vi "ATE_ops_cal.vi"() -> ()   [LabVIEW 2012]
doc: "Use this template to build a producer/consumer design pattern with events to produce queue items. Use this design pattern instead of the User Interface Event Handler pattern for user interfaces when you want to execute code asynchronously in response to an event without slowing the user interface responsiveness."
uses:
  Rvp8PowerData.ctl
  <vilib>/Analysis/NI_AALPro.lvlib
panel:
  in  "ABORT":bool
  in  "READY":bool
  out "Instructions":string="rvp8 calibration vi\n\n1 - Disable or turn off transmitter\n2 - Stow Antenna (point vertically)\n3 - Start the labview program by clicking the Run arrow\n     (left most button under  drop down menues)\n     start cycle time about 35 seconds\n3 - Wait for the red 'BUSY' light to change to green 'READY'\n     The 'active' controls on the control tab are the 'TsPring/TsGrabber'\n     and the 'Start dBm', 'Step Size' and 'Steps' controls \n4 - Calibrate with the red  'Calibrate' button\n      calibration cycle time is about 5 minutes\n5 - Calibration cycle can be aborted with the 'Abort Cal' button which\n     is visable only during the cal cycle\n6 - exit the program with the red 'EXIT' button\n      exit cycle time about 20 seconds\n\nHints:\nWait for the green 'READY' light before clicking buttons"
  out "70dB\nAttenuators":bool[](array[boolean])
  out "70 Verfied":bool
  out "121dB\nAttenuators":bool[](array[boolean])
  out "121 Verified":bool
  in  "Configuration 1":bool
  out "Cal Output File":path
  out "Cal differences":cluster{dbl[], dbl[]}[](graph)
  out "RVP8 calibration":cluster{dbl[], dbl[]}[](graph)
  out "Cal file name":string
  in  "Cal data directory":string="/home/spol/projDir/data/cal/ate/rvp8_cal"
  in  "Set SigGen":bool
  in  "Initialize":bool
  in  "70 dB":bool
  in  "121 dB":bool
  in  "Switches":bool
  in  "Calibrate":bool
  in  "Stop":bool
  in  "ATE TABS":enum32{"Status", "Controls"}(tab)=enum."Controls"
  out "ATE Switch Status":T1
  out "RVP8 Power":T2 {"time" format="%<%H:%M:%S\n%Y/%m/%d>T"}
  out "Signal Generator Status":T3={"Frequency (GHz)"=0.0, "RF Power (dBm)"=0.0, "RF Power"=TRUE} {"RF Power (dBm)" format="%.2g"}
  in  "Start dBm":dbl=-14.0 min=-100.0 max=14.0 step=1.0
  in  "Steps":i32=64
  in  "Steps Size":dbl=2.0 min=0.1 max=10.0 step=0.1 format="%.1g"
  in  "121 dB Atten":i32=121 min=0 max=121 step=1
  in  "70 dB Attn":i32=70 min=0 max=70 step=10
  in  "ATE Switches":T4={"Reversing Switch"=enum."Normal Function", "IO Switch #1 Input"=enum."NONE", "IO Switch #1 Output"=enum."NONE", "IO Switch #2 Input"=enum."NONE", "IO Switch #2 Output"=enum."NONE", "Signal Out Input"=enum."NONE", "Signal Out Output"=enum."NONE", "Signal Source Input"=enum."NONE", "Signal Source Output"=enum."NONE", "Power Meter Switch Input"=enum."NONE", "Pouer Meter Switch Output"=enum."NONE", "Amplifier Switch"=enum."Include Amp"}
  in  "DataSource":bool=TRUE
  out "P-State":string
  out "C-State":string
  in  "BUSY":bool
  # "ATE ops cal Program"
  # "10 dB"
  # "20 dB"
  # "40 dB"
  # "1 dB"
  # "2 dB"
  # "4 dB"
  # "4 dB"
  # "10 dB"
  # "20 dB"
  # "40 dB"
  # "40 dB"
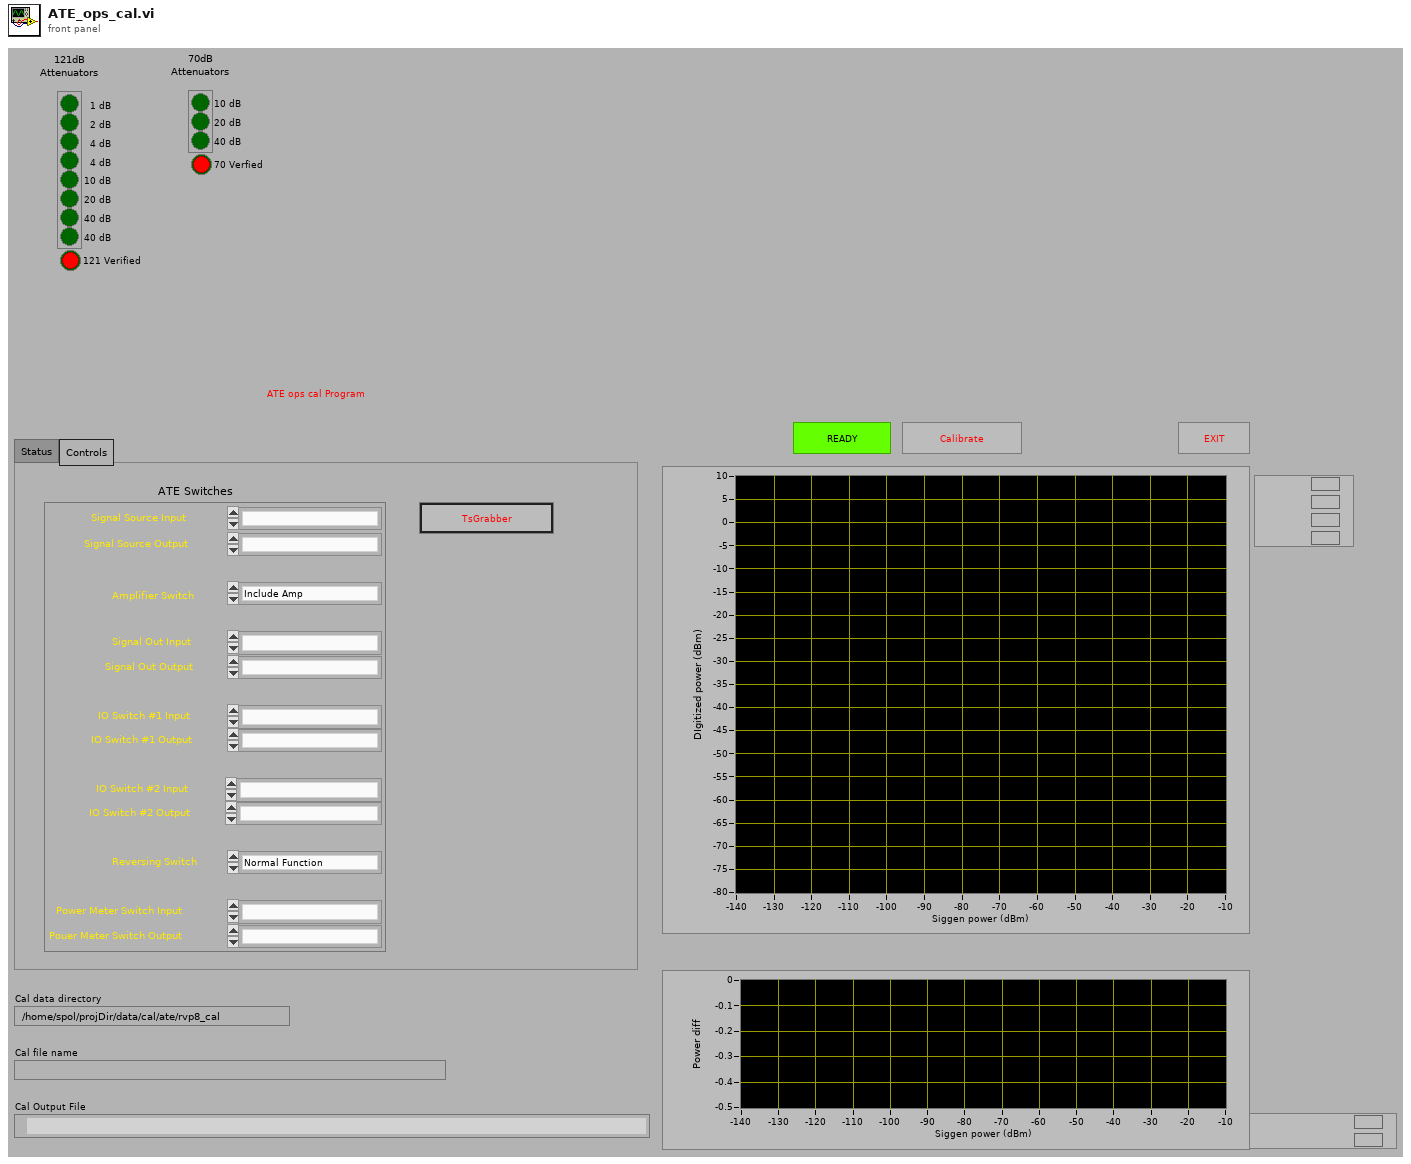
[diagram p1: front panel]
types:
  T1 = cluster{"Reversing Switch ":bool, "IO Switch #1":bool, "IO Switch #2":bool, "Signal Out":bool, "Signal Source":bool, "Power Meter":bool, "Amp By Pass":bool}
  T2 = typedef "Rvp8PowerData.ctl" = cluster{"success":bool, "time":dbl, "el":dbl, "az":dbl, "dbm0":dbl, "dbm1":dbl, "dbmHc":dbl, "dbmHx":dbl, "dbmVc":dbl, "dbmVx":dbl}
  T3 = cluster{"Frequency (GHz)":dbl, "RF Power (dBm)":dbl, "RF Power":bool}
  T4 = cluster{"Reversing Switch":enum16{"Normal Function", "Reversing Function"}, "IO Switch #1 Input":enum16{"NONE", "AHR (J2)", "Splitter", "Signal Out Switch (S3)", "Reversing Switch"}, "IO Switch #1 Output":enum16{"NONE", "AHR (J2)", "Delay Device (S4)", "Power Meter Switch (S5)", "Reversing Switch"}, "IO Switch #2 Input":enum16{"NONE", "AVR (J3)", "Splitter", "Signal Out Switch (S3)", " 2W Term (TM1)", "Reversing Switch"}, "IO Switch #2 Output":enum16{"NONE", "AVR (J3)", "Signal Out Switch (S3)", "Power Meter Switch (S5)", "Reversing Switch", "2W Term (TM1)"}, "Signal Out Input":enum16{"NONE", "Amp Bypass Switch (S6)", "IO Switch #1 (S1)", "IO Switch #2 (S2)", "2W Term (TM3)"}, "Signal Out Output":enum16{"NONE", "2 Watt Term (TM3)", "Splitter", "Power Meter Switch (S5)"}, "Signal Source Input":enum16{"NONE", "Delay Device", "Signal Generator (J7)", "Inside Noise Box NF (J5)", "2W Term (TM3)"}, "Signal Source Output":enum16{"NONE", "Amp Bypass Switch", "Test Pulse Generator", "Power Meter Switch (S5)"}, "Power Meter Switch Input":enum16{"NONE", "IO Switch #1 (S1)", "Signal Source Switch (S4)", "Signal Out Switch (S3)", "IO Switch #2 (S2)", "TXH-TXV Switch (J8)"}, "Pouer Meter Switch Output":enum16{"NONE", "Power Meter (J6)"}, "Amplifier Switch":enum16{"Bypass Amp", "Include Amp"}}
  T5 = cluster{"Frequency (GHz)":dbl, "RF Power (dBm)":dbl, "RF ON/OFF":bool}
  T6 = enum16{"open", "replace", "create", "open or create", "replace or create", "replace or create with confirmation"}
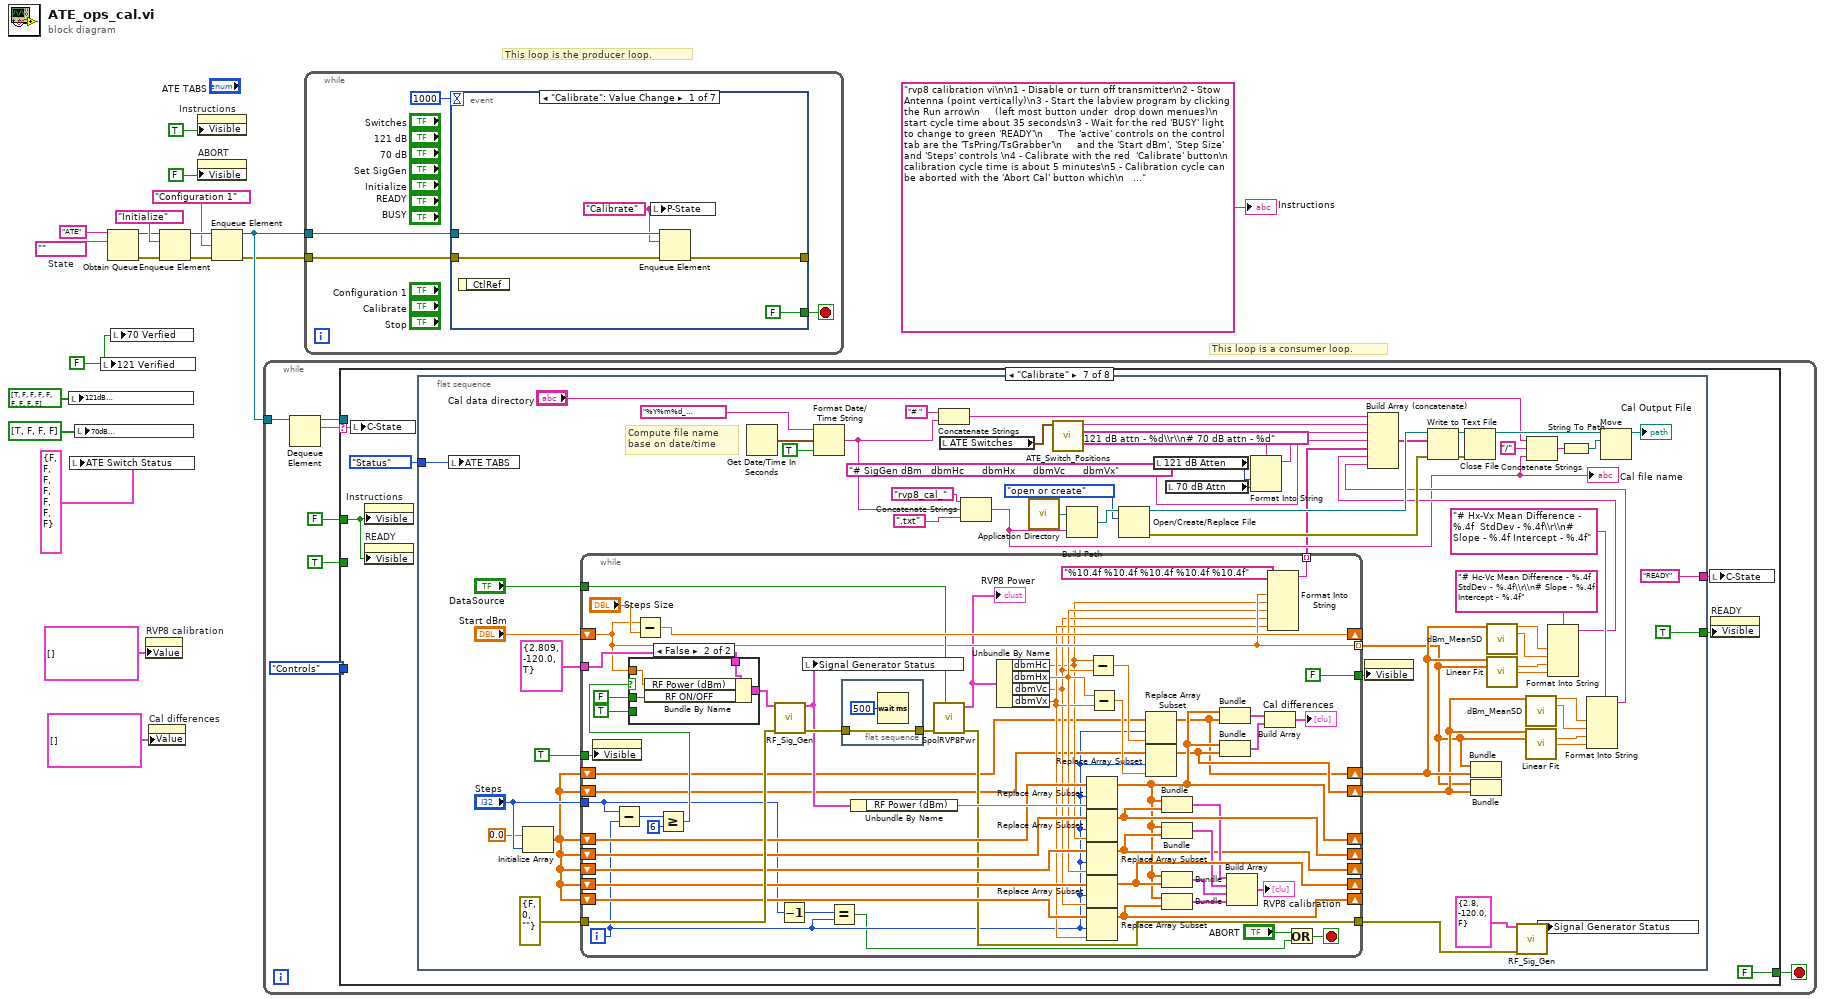
[diagram p0: block diagram]
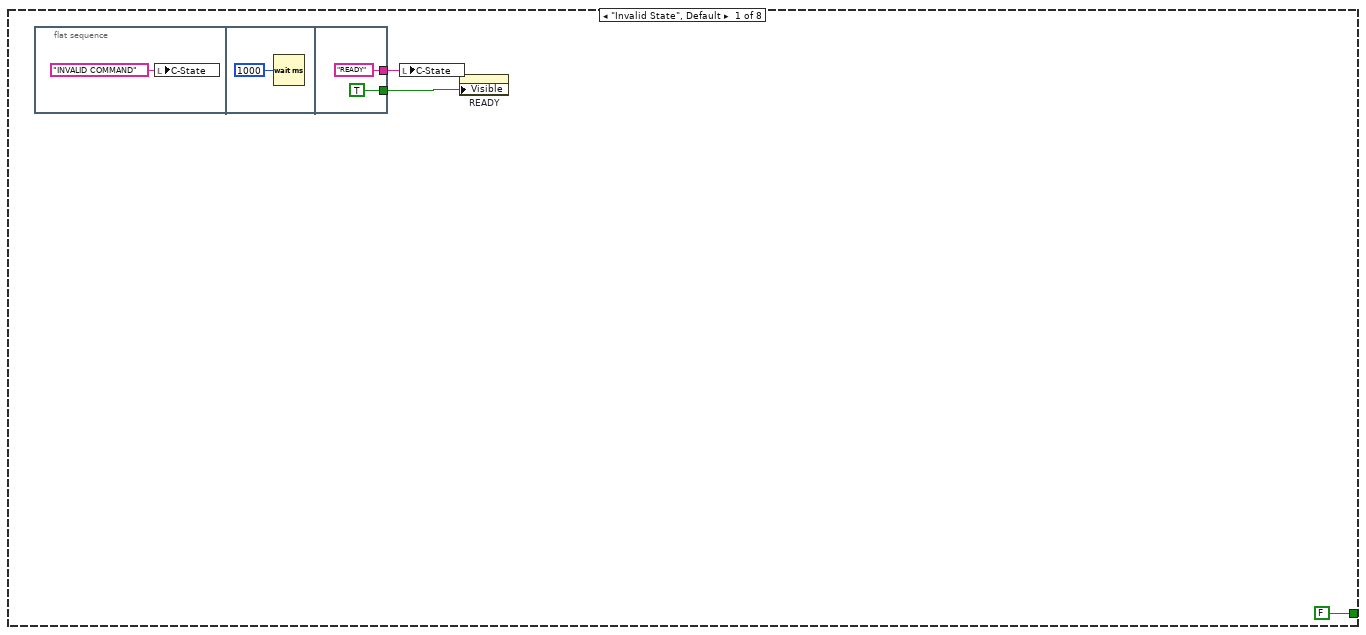
[diagram p2: hidden frame]
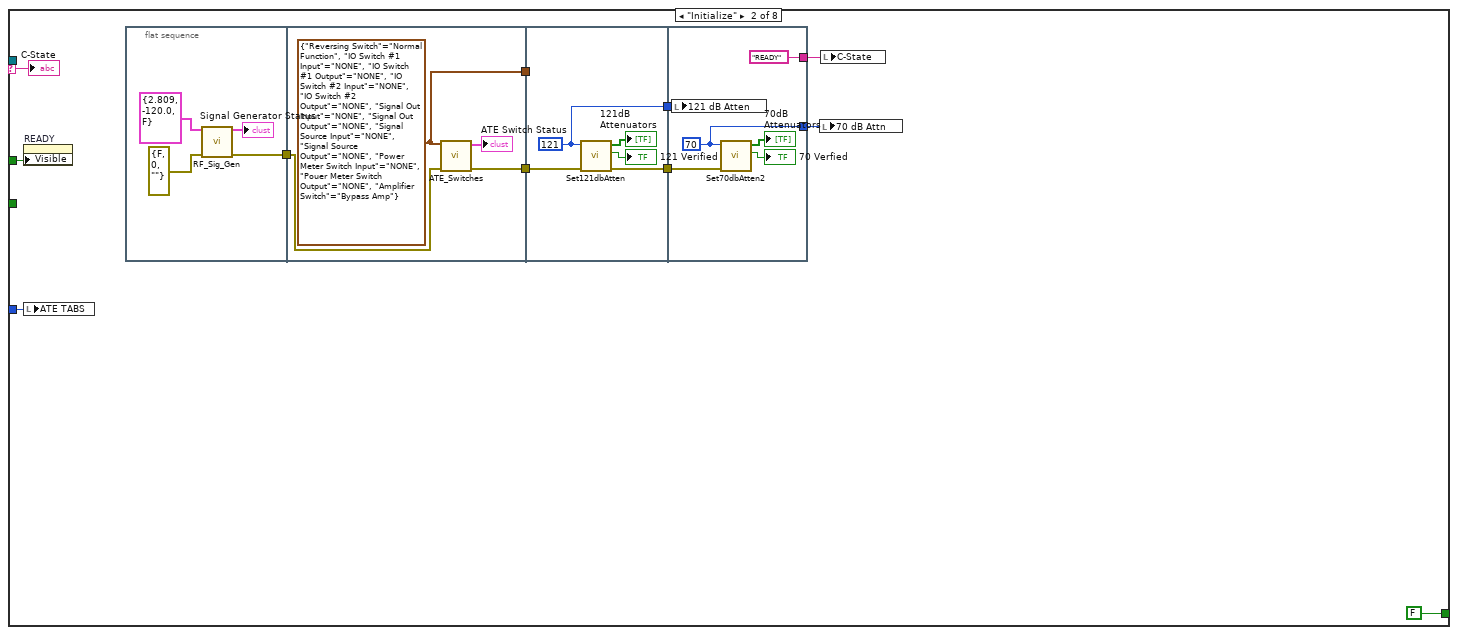
[diagram p3: hidden frame]
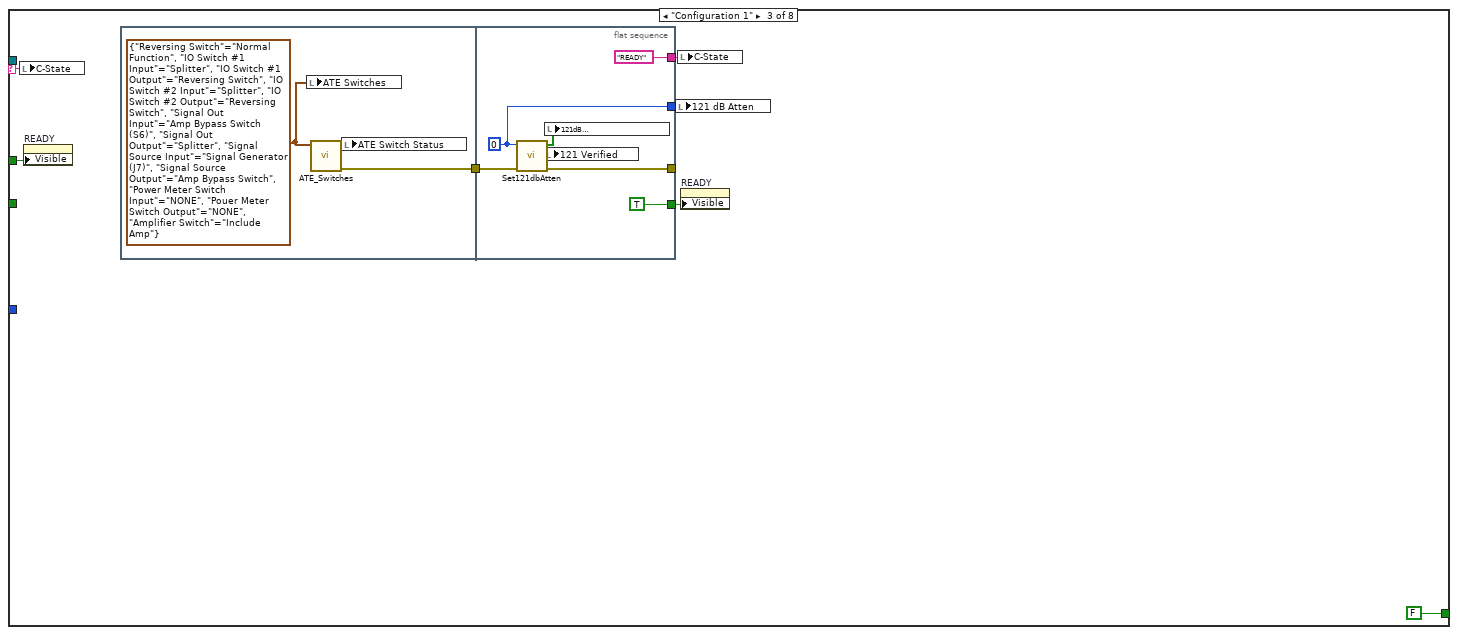
[diagram p4: hidden frame]
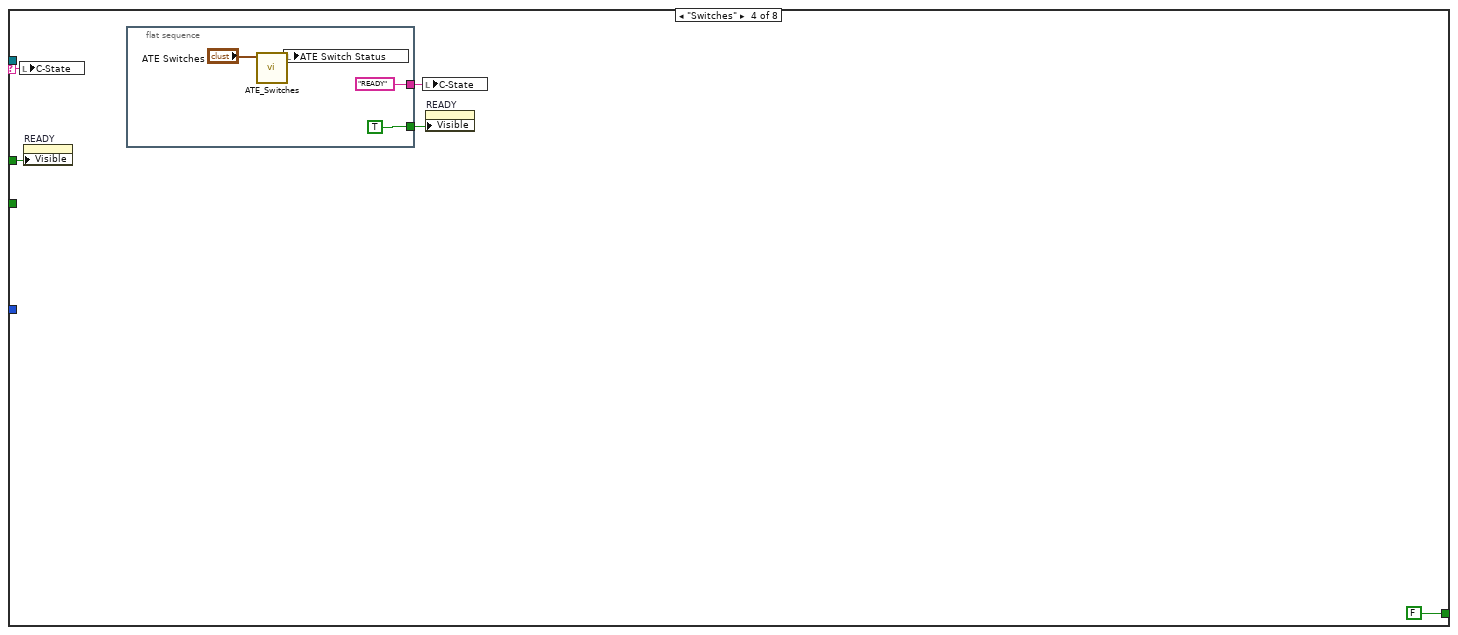
[diagram p5: hidden frame]
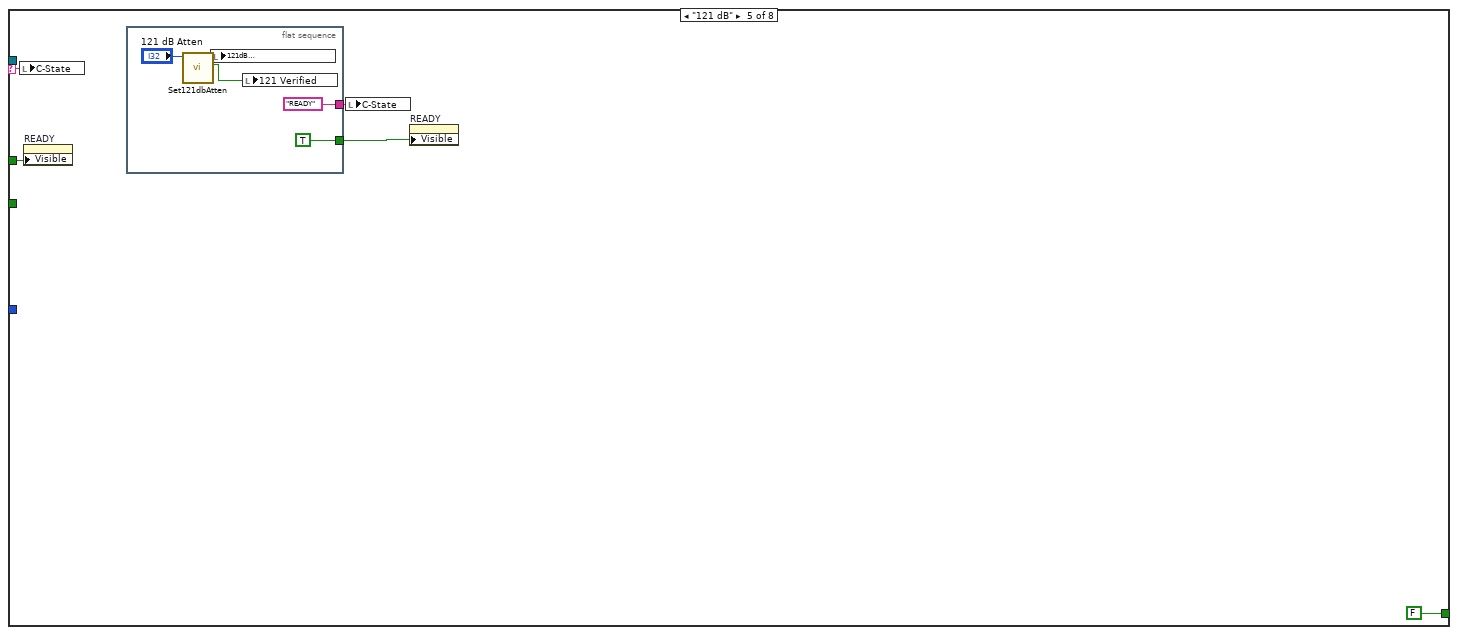
[diagram p6: hidden frame]
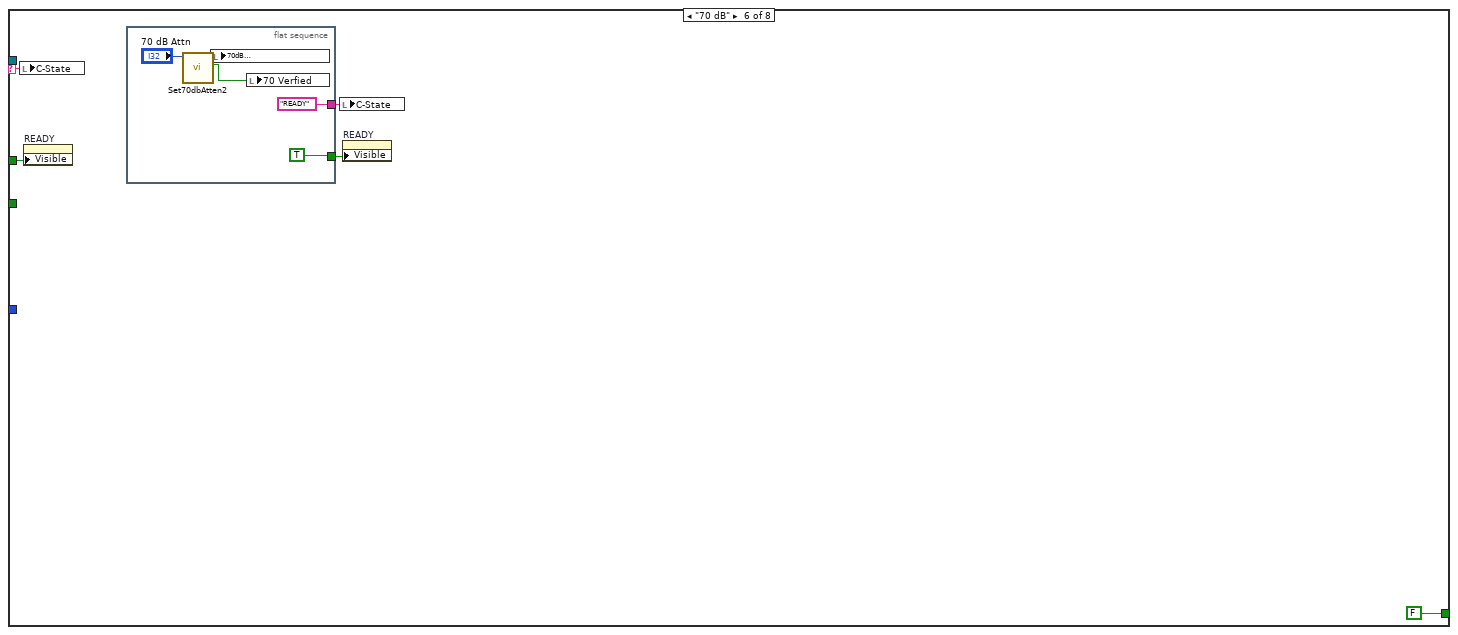
[diagram p7: hidden frame]
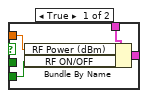
[diagram p8: hidden frame]
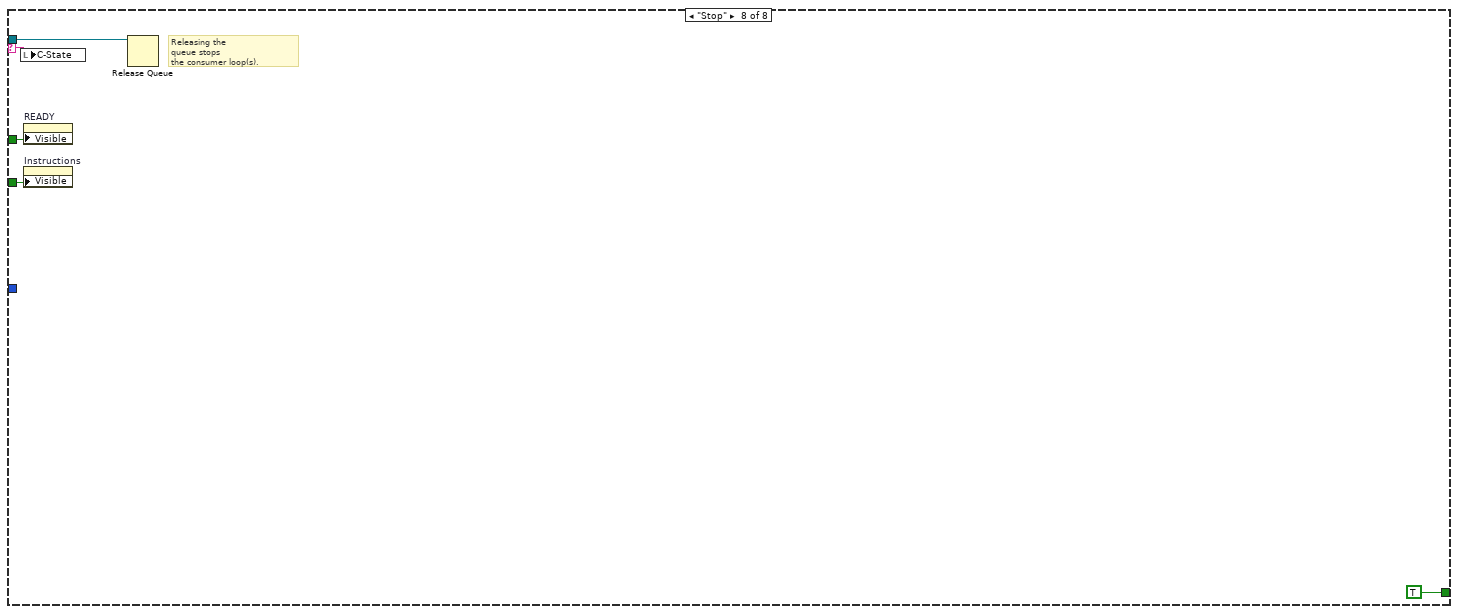
[diagram p9: hidden frame]
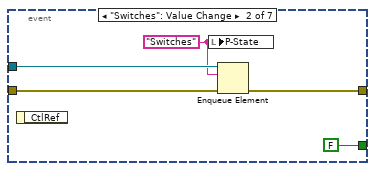
[diagram p10: hidden frame]
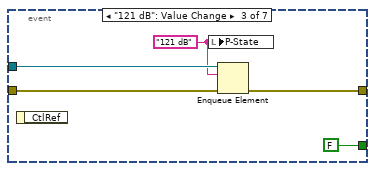
[diagram p11: hidden frame]
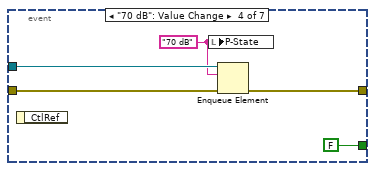
[diagram p12: hidden frame]
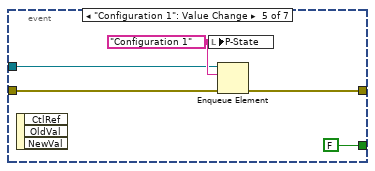
[diagram p13: hidden frame]
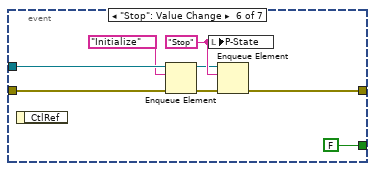
[diagram p14: hidden frame]
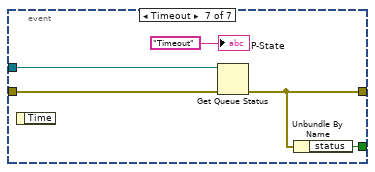
[diagram p15: hidden frame]
diagram:
  w4 = FALSE ("70 Verfied")
  w19 = ""  # State
  # "This loop is the producer loop."
  # "This loop is a consumer loop."
  n1 = local write "121dB\nAttenuators"(bool[] [TRUE, FALSE, FALSE, FALSE, FALSE, FALSE, FALSE, FALSE, FALSE] ("121dB\nAttenuators")) -> ()
  n2 = local write "ATE Switch Status"(T1 {"Reversing Switch "=FALSE, "IO Switch #1"=FALSE, "IO Switch #2"=FALSE, "Signal Out"=FALSE, "Signal Source"=FALSE, "Power Meter"=FALSE, "Amp By Pass"=FALSE} ("ATE Switch Status")) -> ()
  n3 = local write "70dB\nAttenuators"(bool[] [TRUE, FALSE, FALSE, FALSE] ("70dB\nAttenuators")) -> ()
  n4 = local write "121 Verified"(w4) -> ()
  n5 = Obtain Queue(name (unnamed)="ATE", element data type=w19) -> (queue out=w16:refnum<queue>, error out=w14:errorcluster)  [unwired: 3 in, 1 out]
  n6 = local write "70 Verfied"(w4) -> ()
  n7 = property on="RVP8 calibration" class="XYGraph (strict)"("Value"=cluster{dbl[], dbl[]}[] [] ("RVP8 calibration")) -> ()  [unwired: 2 in, 2 out]
  n8 = property on="Cal differences" class="XYGraph (strict)"("Value"=cluster{dbl[], dbl[]}[] [] ("Cal differences")) -> ()  [unwired: 2 in, 2 out]
  n9 = Enqueue Element(queue=w16, element="Initialize", error in (no error)=w14) -> (queue out=w15:refnum<queue>, error out=w9:errorcluster)  [unwired: 1 in, 1 out]
  n10 = property on="Instructions" class="Str"("Visible"=TRUE) -> ()  [unwired: 2 in, 2 out]
  n11 = property on="ABORT" class="Bool"("Visible"=FALSE) -> ()  [unwired: 2 in, 2 out]
  n12 = Enqueue Element(queue=w15, element="Configuration 1", error in (no error)=w9) -> (queue out=w10:refnum<queue>, error out=w8:errorcluster)  [unwired: 1 in, 1 out]
  n13 = while {
    tunnel: w10 -> [w26]
    stop <- w23 stop-if-true
    n14 = Dequeue Element(queue=w26) -> (queue out=w24:refnum<queue>, element=w25:string)  [unwired: 2 in, 2 out]
    n15 = case shown="\"Calibrate\"" w25 {
      selector: w25 -> [_ w43 w66 w85 w93 w103 w114 w246]
      tunnel: w24 -> [_ _ _ _ _ _ _ w245]
      tunnel: [FALSE FALSE FALSE FALSE FALSE FALSE FALSE TRUE] -> w23
      tunnel: FALSE ("Visible") -> [_ w35 w65 w82 w91 w101 w112 w244]
      tunnel: TRUE ("Visible") -> [_ _ _ _ _ _ _ w243]
      tunnel: enum32{"Status", "Controls"}."Controls" ("ATE TABS") -> [_ w34 _ _ _ _ _ _]
      frame "Invalid State", Default {
        n16 = flat-sequence {
          tunnel: ["READY" ("element")] -> w28
          tunnel: [TRUE ("Visible")] -> w27
          frame #0 {
            n17 = local write "C-State"("INVALID COMMAND" ("C-State")) -> ()
          }
          frame #1 {
            n18 = Wait (ms)(milliseconds to wait=u32 1000) -> ()  [unwired: 1 out]
          }
          frame #2 {
          }
        }
        n19 = local write "C-State"(w28) -> ()
        n20 = property on="READY" class="Bool"("Visible"=w27) -> ()  [unwired: 2 in, 2 out]
      }
      frame "Initialize" {
        n21 = property on="READY" class="Bool"("Visible"=w35) -> ()  [unwired: 2 in, 2 out]
        n22 = local write "ATE TABS"(w34) -> ()
        n23 = flat-sequence {
          tunnel: [w45] -> w37
          tunnel: [w50] -> w40
          tunnel: w37 -> [w51]
          tunnel: [w49] -> w36
          tunnel: w40 -> [w56]
          tunnel: [w55] -> w41
          tunnel: [w54] -> w39
          tunnel: w36 -> [_]
          tunnel: ["READY" ("element")] -> w42
          tunnel: w41 -> [w62]
          tunnel: w39 -> [w60]
          tunnel: [w59] -> w38
          frame #0 {
            n24 = call "RF_Sig_Gen.vi"("Signal Generator Control"=T5 {"Frequency (GHz)"=2.809, "RF Power (dBm)"=-120.0, "RF ON/OFF"=FALSE}, "error in"=errorcluster {"status"=FALSE, "code"=0, "source"=""}) -> ("Signal Generator Status"=→"Signal Generator Status":T3, "Sig Gen Errors"=w45:errorcluster)  [unwired: 12 in]
          }
          frame #1 {
            w49 = T4 {"Reversing Switch"=enum."Normal Function", "IO Switch #1 Input"=enum."NONE", "IO Switch #1 Output"=enum."NONE", "IO Switch #2 Input"=enum."NONE", "IO Switch #2 Output"=enum."NONE", "Signal Out Input"=enum."NONE", "Signal Out Output"=enum."NONE", "Signal Source Input"=enum."NONE", "Signal Source Output"=enum."NONE", "Power Meter Switch Input"=enum."NONE", "Pouer Meter Switch Output"=enum."NONE", "Amplifier Switch"=enum."Bypass Amp"} ("ATE Switches")
            n25 = call "ATE_Switches.vi"("error in"=w51, "ATE Switches"=w49) -> ("Switch Errors"=w50:errorcluster, "ATE Switch Status"=→"ATE Switch Status":T1)  [unwired: 8 in]
          }
          frame #2 {
            w54 = 121 ("Attenuation (dB)")
            n26 = call "Set121dbAtten.vi"("error in (no error)"=w56, "Attenuation (dB)"=w54) -> ("error out"=w55:errorcluster, "Verfied"=→"121 Verified":bool, "Active Attenuators"=→"121dB\nAttenuators":bool[])  [unwired: 7 in]
          }
          frame #3 {
            w59 = 70 ("Attenuation (dB)")
            n27 = local write "121 dB Atten"(w60) -> ()
            n28 = call "Set70dbAtten2.vi"("error in (no error)"=w62, "Attenuation (dB)"=w59) -> ("Verfied"=→"70 Verfied":bool, "Active Attenuators"=→"70dB\nAttenuators":bool[])  [unwired: 7 in, 1 out]
          }
        }
        n29 = local write "70 dB Attn"(w38) -> ()
        n30 = local write "C-State"(w42) -> ()
        "C-State" <- w43
      }
      frame "Configuration 1" {
        n31 = local write "C-State"(w66) -> ()
        n32 = property on="READY" class="Bool"("Visible"=w65) -> ()  [unwired: 2 in, 2 out]
        n33 = flat-sequence {
          tunnel: [w73] -> w69
          tunnel: w69 -> [w80]
          tunnel: [w75] -> w68
          tunnel: ["READY" ("element")] -> w67
          tunnel: [w78] -> _
          tunnel: [TRUE ("Visible")] -> w64
          frame #0 {
            w71 = T4 {"Reversing Switch"=enum."Normal Function", "IO Switch #1 Input"=enum."Splitter", "IO Switch #1 Output"=enum."Reversing Switch", "IO Switch #2 Input"=enum."Splitter", "IO Switch #2 Output"=enum."Reversing Switch", "Signal Out Input"=enum."Amp Bypass Switch (S6)", "Signal Out Output"=enum."Splitter", "Signal Source Input"=enum."Signal Generator (J7)", "Signal Source Output"=enum."Amp Bypass Switch", "Power Meter Switch Input"=enum."NONE", "Pouer Meter Switch Output"=enum."NONE", "Amplifier Switch"=enum."Include Amp"} ("ATE Switches")
            n34 = local write "ATE Switches"(w71) -> ()
            n35 = call "ATE_Switches.vi"("ATE Switches"=w71) -> ("Switch Errors"=w73:errorcluster, "ATE Switch Status"=w72:T1)  [unwired: 9 in]
            n36 = local write "ATE Switch Status"(w72) -> ()
          }
          frame #1 {
            w75 = 0 ("Attenuation (dB)")
            n37 = call "Set121dbAtten.vi"("error in (no error)"=w80, "Attenuation (dB)"=w75) -> ("error out"=w78:errorcluster, "Verfied"=w76:bool, "Active Attenuators"=w77:bool[])  [unwired: 7 in]
            n38 = local write "121 Verified"(w76) -> ()
            n39 = local write "121dB\nAttenuators"(w77) -> ()
          }
        }
        n40 = local write "121 dB Atten"(w68) -> ()
        n41 = local write "C-State"(w67) -> ()
        n42 = property on="READY" class="Bool"("Visible"=w64) -> ()  [unwired: 2 in, 2 out]
      }
      frame "Switches" {
        n43 = local write "C-State"(w85) -> ()
        n44 = property on="READY" class="Bool"("Visible"=w82) -> ()  [unwired: 2 in, 2 out]
        n45 = flat-sequence {
          tunnel: ["READY" ("element")] -> w83
          tunnel: [TRUE ("Visible")] -> w81
          frame #0 {
            n46 = call "ATE_Switches.vi"("ATE Switches"="ATE Switches") -> ("ATE Switch Status"=w88:T1)  [unwired: 9 in, 1 out]
            n47 = local write "ATE Switch Status"(w88) -> ()
          }
        }
        n48 = local write "C-State"(w83) -> ()
        n49 = property on="READY" class="Bool"("Visible"=w81) -> ()  [unwired: 2 in, 2 out]
      }
      frame "121 dB" {
        n50 = local write "C-State"(w93) -> ()
        n51 = property on="READY" class="Bool"("Visible"=w91) -> ()  [unwired: 2 in, 2 out]
        n52 = flat-sequence {
          tunnel: ["READY" ("element")] -> w92
          tunnel: [TRUE ("Visible")] -> w90
          frame #0 {
            n53 = call "Set121dbAtten.vi"("Attenuation (dB)"="121 dB Atten") -> ("Verfied"=w96:bool, "Active Attenuators"=w98:bool[])  [unwired: 8 in, 1 out]
            n54 = local write "121dB\nAttenuators"(w98) -> ()
            n55 = local write "121 Verified"(w96) -> ()
          }
        }
        n56 = local write "C-State"(w92) -> ()
        n57 = property on="READY" class="Bool"("Visible"=w90) -> ()  [unwired: 2 in, 2 out]
      }
      frame "70 dB" {
        n58 = local write "C-State"(w103) -> ()
        n59 = property on="READY" class="Bool"("Visible"=w101) -> ()  [unwired: 2 in, 2 out]
        n60 = flat-sequence {
          tunnel: ["READY" ("element")] -> w102
          tunnel: [TRUE ("Visible")] -> w100
          frame #0 {
            n61 = call "Set70dbAtten2.vi"("Attenuation (dB)"="70 dB Attn") -> ("Verfied"=w106:bool, "Active Attenuators"=w108:bool[])  [unwired: 8 in, 1 out]
            n62 = local write "70dB\nAttenuators"(w108) -> ()
            n63 = local write "70 Verfied"(w106) -> ()
          }
        }
        n64 = local write "C-State"(w102) -> ()
        n65 = property on="READY" class="Bool"("Visible"=w100) -> ()  [unwired: 2 in, 2 out]
      }
      frame "Calibrate" {
        n66 = local write "C-State"(w114) -> ()
        n67 = property on="Instructions" class="Str"("Visible"=w112) -> ()  [unwired: 2 in, 2 out]
        n68 = property on="READY" class="Bool"("Visible"=w112) -> ()  [unwired: 2 in, 2 out]
        n69 = flat-sequence {
          tunnel: ["READY" ("element")] -> w113
          tunnel: [TRUE ("Visible")] -> w111
          tunnel: enum32{"Status", "Controls"}."Status" ("ATE TABS") -> [w121]
          frame #0 {
            # "Compute file name base on date/time"
            n70 = local write "ATE TABS"(w121) -> ()
            n71 = Initialize Array(0.0 ("element"), "Steps") -> (w120:dbl[])
            n72 = while {
              shift-right: [w226] -> _
              shift-left: "Start dBm" -> [w223]
              tunnel: errorcluster {"status"=FALSE, "code"=0, "source"=""} ("error out") -> [w217]
              tunnel: [w223] -> w123 mode=indexing
              tunnel: [w232] -> w126 mode=indexing
              tunnel: T5 {"Frequency (GHz)"=2.809, "RF Power (dBm)"=-120.0, "RF ON/OFF"=TRUE} ("Signal Generator Control") -> [w231]
              tunnel: [w195] -> w157
              tunnel: "DataSource" -> [w225]
              tunnel: "Steps" -> [w180]
              shift-right: [w194] -> _
              shift-left: w120 -> [w209]
              shift-right: [w206] -> _
              shift-left: w120 -> [w213]
              shift-right: [w196] -> _
              shift-left: w120 -> [w214]
              shift-right: [w208] -> _
              shift-left: w120 -> [w215]
              shift-right: [w207] -> _
              shift-left: w120 -> [w216]
              shift-right: [w190] -> w149
              shift-left: w120 -> [w188]
              shift-right: [w191] -> w148
              shift-left: w120 -> [w189]
              tunnel: [FALSE ("Visible")] -> w119
              tunnel: TRUE ("Visible") -> [w177]
              i -> [w182]
              stop <- w184 stop-if-true
              n73 = property on="ABORT" class="Bool"("Visible"=w177) -> ()  [unwired: 2 in, 2 out]
              n74 = Subtract(x=w180, y=w182) -> (x-y=w218:i32)
              n75 = Subtract(x=w223, y="Steps Size") -> (x-y=w226:dbl)
              n76 = Greater Or Equal?(x=w218, y=6) -> (x >= y?=w220:bool)
              n77 = case shown="False" w220 {
                tunnel: w231 -> [w236 w240]
                tunnel: [w235 w239] -> w227
                tunnel: w223 -> [w234 w238]
                tunnel: FALSE ("70 Verfied") -> [_ w237]
                tunnel: TRUE ("70 Verfied") -> [w233 _]
                frame True {
                  n78 = Bundle By Name(cluster=w236, "RF Power (dBm)"=w234, "RF ON/OFF"=w233) -> (w235:T5)
                }
                frame False {
                  n79 = Bundle By Name(cluster=w240, "RF Power (dBm)"=w238, "RF ON/OFF"=w237) -> (w239:T5)
                }
              }
              n80 = call "RF_Sig_Gen.vi"("Signal Generator Control"=w227, "error in"=w217) -> ("Signal Generator Status"=w211:T3, "Sig Gen Errors"=w230:errorcluster)  [unwired: 12 in]
              n81 = Decrement(x=w180) -> (x-1=w181:i32)
              n82 = local write "Signal Generator Status"(w211) -> ()
              n83 = Equal?(x=w181, y=w182) -> (x = y?=w179:bool)
              n84 = flat-sequence {
                tunnel: w230 -> [w242]
                tunnel: [w242] -> w229
                frame #0 {
                  n85 = Wait (ms)(milliseconds to wait=u32 500) -> ()  [unwired: 1 out]
                }
              }
              n86 = Unbundle By Name(w211) -> ("RF Power (dBm)"=w210:dbl)
              n87 = call "SpolRVP8Pwr.vi"("DataSource"=w225, "error in (no error)"=w229) -> ("Comm error"=w195:errorcluster, "RVP8_power"=w212:T2)  [unwired: 6 in, 2 out]
              "RVP8 Power" <- w212
              n88 = Unbundle By Name(w212) -> ("dbmHc"=w197:dbl, "dbmHx"=w200:dbl, "dbmVc"=w198:dbl, "dbmVx"=w199:dbl)
              n89 = Replace Array Subset(array=w209, new element=w210, index=w182) -> (w194:dbl[])
              n90 = Replace Array Subset(array=w213, new element=w197, index=w182) -> (w206:dbl[])
              n91 = Replace Array Subset(array=w214, new element=w200, index=w182) -> (w196:dbl[])
              n92 = Replace Array Subset(array=w215, new element=w198, index=w182) -> (w208:dbl[])
              n93 = Replace Array Subset(array=w216, new element=w199, index=w182) -> (w207:dbl[])
              n94 = Subtract(x=w197, y=w198) -> (x-y=w193:dbl)
              n95 = Subtract(x=w200, y=w199) -> (x-y=w192:dbl)
              n96 = Replace Array Subset(array=w188, new element=w193, index=w182) -> (w190:dbl[])
              n97 = Replace Array Subset(array=w189, new element=w192, index=w182) -> (w191:dbl[])
              n98 = Bundle(w194, w206) -> (w202:cluster{dbl[], dbl[]})  [unwired: 1 in]
              n99 = Bundle(w194, w196) -> (w203:cluster{dbl[], dbl[]})  [unwired: 1 in]
              n100 = Bundle(w194, w208) -> (w204:cluster{dbl[], dbl[]})  [unwired: 1 in]
              n101 = Bundle(w194, w207) -> (w205:cluster{dbl[], dbl[]})  [unwired: 1 in]
              n102 = Bundle(w194, w190) -> (w186:cluster{dbl[], dbl[]})  [unwired: 1 in]
              n103 = Bundle(w194, w191) -> (w187:cluster{dbl[], dbl[]})  [unwired: 1 in]
              n104 = Build Array(w202, w203, w204, w205) -> (→"RVP8 calibration":cluster{dbl[], dbl[]}[])
              n105 = Build Array(w186, w187) -> (→"Cal differences":cluster{dbl[], dbl[]}[])
              n106 = Format Into String(format string="%10.4f %10.4f %10.4f %10.4f %10.4f", w223, w197, w200, w198, w199) -> (resulting string=w232:string)  [unwired: 2 in, 1 out]
              n107 = Or(x="ABORT", y=w179) -> (x .or. y?=w184:bool)
            }
            n108 = Get Date/Time In Seconds() -> (seconds since 1Jan1904=w171:timestamp)
            n109 = Format Date/Time String(time format string (%c)="%Y%m%d_%H%M%S", seconds (now)=w171, UTC format=TRUE) -> (date/time string=w128:string)
            n110 = Concatenate Strings("# " ("string"), w128) -> (w142:string)
            n111 = local read "ATE Switches"() -> (w135:T4)
            n112 = Concatenate Strings("rvp8_cal_", w128, ".txt") -> (w127:string)
            "Cal file name" <- w127
            n113 = call <vilib>:"Application Directory.vi"() -> ("Application Directory"=w132:path)
            n114 = call "ATE_Switch_Positions.vi"("ATE Switches"=w135) -> ("ATE Switch/Position"=w141:string)  [unwired: 10 in]
            n115 = Build Path(base path=w132, name or relative path=w127) -> (appended path=w168:path)
            n116 = Open/Create/Replace File(file path (use dialog)=w168, operation (0:open)=T6."open or create") -> (refnum out=w167:refnum<file>, error out=w166:errorcluster)  [unwired: 4 in, 1 out]
            n117 = local read "121 dB Atten"() -> (w154:i32)
            n118 = local read "70 dB Attn"() -> (w153:i32)
            n119 = Format Into String(format string="# 121 dB attn - %d\\r\\n# 70 dB attn - %d", w154, w153) -> (resulting string=w140:string)  [unwired: 2 in, 1 out]
            n120 = property on="ABORT" class="Bool"("Visible"=w119) -> ()  [unwired: 2 in, 2 out]
            n121 = Bundle(w123, w149) -> ()  [unwired: 1 in, 1 out]
            n122 = Bundle(w123, w148) -> ()  [unwired: 1 in, 1 out]
            n123 = call "dBm_MeanSD.vi"("dBm array"=w149) -> ("dBm mean"=w152:dbl, "Std Dev"=w116:dbl)  [unwired: 13 in]
            n124 = call <vilib>:"Linear Fit.vi"("Y"=w149, "X"=w123) -> ("slope"=w151:dbl, "intercept"=w150:dbl)  [unwired: 9 in, 3 out]
            n125 = call "RF_Sig_Gen.vi"("Signal Generator Control"=T5 {"Frequency (GHz)"=2.8, "RF Power (dBm)"=-120.0, "RF ON/OFF"=FALSE}, "error in"=w157) -> ("Signal Generator Status"=w158:T3)  [unwired: 12 in, 1 out]
            n126 = call "dBm_MeanSD.vi"("dBm array"=w148) -> ("dBm mean"=w147:dbl, "Std Dev"=w117:dbl)  [unwired: 13 in]
            n127 = call <vilib>:"Linear Fit.vi"("Y"=w148, "X"=w123) -> ("slope"=w146:dbl, "intercept"=w145:dbl)  [unwired: 9 in, 3 out]
            n128 = Concatenate Strings("Cal data directory", "/" ("string"), w127) -> (w162:string)
            n129 = local write "Signal Generator Status"(w158) -> ()
            n130 = Format Into String(format string="# Hc-Vc Mean Difference - %.4f  StdDev - %.4f\\r\\n# Slope - %.4f Intercept - %.4f", w152, w116, w151, w150) -> (resulting string=w131:string)  [unwired: 2 in, 1 out]
            n131 = String To Path(string=w162) -> (path=w160:path)
            n132 = Format Into String(format string="# Hx-Vx Mean Difference - %.4f  StdDev - %.4f\\r\\n# Slope - %.4f Intercept - %.4f", w147, w117, w146, w145) -> (resulting string=w130:string)  [unwired: 2 in, 1 out]
            n133 = Build Array (concatenate)(w142, w141, w140, "# SigGen dBm   dbmHc      dbmHx      dbmVc      dbmVx", w126, w131, w130) -> (w156:string[])
            n134 = Write to Text File(file (use dialog)=w167, text=w156, error in=w166) -> (refnum out=w165:refnum<file>, error out=w164:errorcluster)  [unwired: 1 in, 1 out]
            n135 = Close File(refnum=w165, error in=w164) -> (path=w161:path)  [unwired: 1 out]
            n136 = Move(source path=w161, 10:w160) -> (3:→"Cal Output File":path)  [unwired: 3 in, 2 out]
          }
        }
        n137 = local write "C-State"(w113) -> ()
        n138 = property on="READY" class="Bool"("Visible"=w111) -> ()  [unwired: 2 in, 2 out]
      }
      frame "Stop" {
        # "Releasing the\nqueue stops\nthe consumer loop(s)."
        n139 = local write "C-State"(w246) -> ()
        n140 = property on="READY" class="Bool"("Visible"=w244) -> ()  [unwired: 2 in, 2 out]
        n141 = property on="Instructions" class="Str"("Visible"=w243) -> ()  [unwired: 2 in, 2 out]
        n142 = Release Queue(queue=w245) -> ()  [unwired: 2 in, 3 out]
      }
    }
  }
  n143 = while {
    tunnel: w10 -> [w251]
    tunnel: w8 -> [w250]
    stop <- w248 stop-if-true
    n144 = event shown="[0] \"Calibrate\": Value Change" {
      selector: _ -> [_ _ _ _ _ _ _]
      dyn-events: _ -> [_ _ _ _ _ _ _]
      timeout: 1000 -> [_ _ _ _ _ _ _]
      tunnel: w251 -> [w256 w261 w266 w271 w275 w279 w289]
      tunnel: w250 -> [w255 w260 w265 w270 w274 w281 w285]
      tunnel: [w254 w259 w264 w269 w273 w284 w287] -> _
      tunnel: [FALSE FALSE FALSE FALSE FALSE ("status") FALSE w288] -> w248
      event "Calibrate": Value Change {
        w252 = "Calibrate" ("element")
        n145 = event-data() -> ()  [unwired: 1 in, 1 out]
        n146 = local write "P-State"(w252) -> ()
        n147 = Enqueue Element(queue=w256, element=w252, error in (no error)=w255) -> (error out=w254:errorcluster)  [unwired: 1 in, 2 out]
      }
      event "Switches": Value Change {
        w257 = "Switches" ("element")
        n148 = event-data() -> ()  [unwired: 1 in, 1 out]
        n149 = local write "P-State"(w257) -> ()
        n150 = Enqueue Element(queue=w261, element=w257, error in (no error)=w260) -> (error out=w259:errorcluster)  [unwired: 1 in, 2 out]
      }
      event "121 dB": Value Change {
        w262 = "121 dB" ("element")
        n151 = event-data() -> ()  [unwired: 1 in, 1 out]
        n152 = local write "P-State"(w262) -> ()
        n153 = Enqueue Element(queue=w266, element=w262, error in (no error)=w265) -> (error out=w264:errorcluster)  [unwired: 1 in, 2 out]
      }
      event "70 dB": Value Change {
        w267 = "70 dB" ("element")
        n154 = event-data() -> ()  [unwired: 1 in, 1 out]
        n155 = local write "P-State"(w267) -> ()
        n156 = Enqueue Element(queue=w271, element=w267, error in (no error)=w270) -> (error out=w269:errorcluster)  [unwired: 1 in, 2 out]
      }
      event "Configuration 1": Value Change {
        w276 = "Configuration 1" ("element")
        n157 = event-data() -> ()  [unwired: 1 in, 3 out]
        n158 = local write "P-State"(w276) -> ()
        n159 = Enqueue Element(queue=w275, element=w276, error in (no error)=w274) -> (error out=w273:errorcluster)  [unwired: 1 in, 2 out]
      }
      event "Stop": Value Change {
        w282 = "Stop" ("element")
        n160 = event-data() -> ()  [unwired: 1 in, 1 out]
        n161 = Enqueue Element(queue=w279, element="Initialize", error in (no error)=w281) -> (queue out=w278:refnum<queue>, error out=w280:errorcluster)  [unwired: 1 in, 1 out]
        n162 = local write "P-State"(w282) -> ()
        n163 = Enqueue Element(queue=w278, element=w282, error in (no error)=w280) -> (error out=w284:errorcluster)  [unwired: 1 in, 2 out]
      }
      event Timeout {
        n164 = event-data() -> ()  [unwired: 1 in, 1 out]
        n165 = Get Queue Status(queue=w289, error in (no error)=w285) -> (error out=w287:errorcluster)  [unwired: 1 in, 7 out]
        n166 = Unbundle By Name(w287) -> ("status"=w288:bool)
        "P-State" <- "Timeout" ("element")
      }
    }
  }
  "Instructions" <- "rvp8 calibration vi\n\n1 - Disable or turn off transmitter\n2 - Stow Antenna (point vertically)\n3 - Start the labview program by clicking the Run arrow\n     (left most button under  drop down menues)\n     start cycle time about 35 seconds\n3 - Wait for the red 'BUSY' light to change to green 'READY'\n     The 'active' controls on the control tab are the 'TsPring/TsGrabber'\n     and the 'Start dBm', 'Step Size' and 'Steps' controls \n4 - Calibrate with the red  'Calibrate' button\n      calibration cycle time is about 5 minutes\n5 - Calibration cycle can be aborted with the 'Abort Cal' button which\n     is visable only during the cal cycle\n6 - exit the program with the red 'EXIT' button\n      exit cycle time about 20 seconds\n\nHints:\nWait for the green 'READY' light before clicking buttons" ("String")
